vi "generateTimeStamp.vi"(8 "error in (no error)":errorcluster, 11 "FileNeologist in":refnum<class "FileNeologist.lvclass">) -> (0 "error out":errorcluster, 3 "FileNeologist out":refnum<class "FileNeologist.lvclass">)   [LabVIEW 2009, in "Tools.lvlib" / "Filing.lvlib" / "FileNeologist.lvclass"]
uses:
  FileNeologist.lvclass
  FileNeologist.lvclass/FileNeologist.ctl
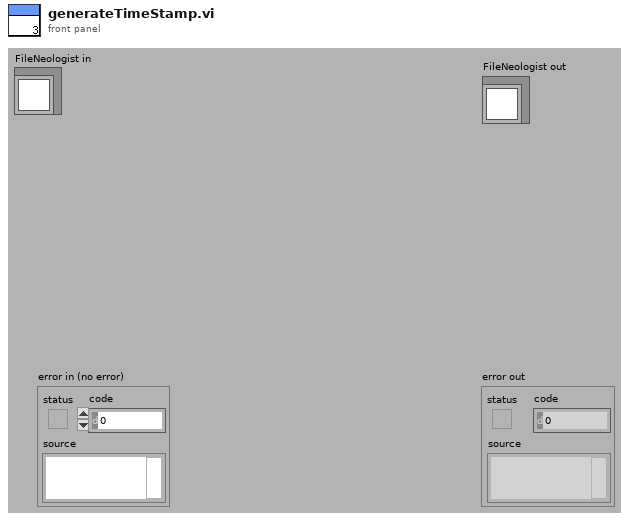
[diagram p1: front panel]
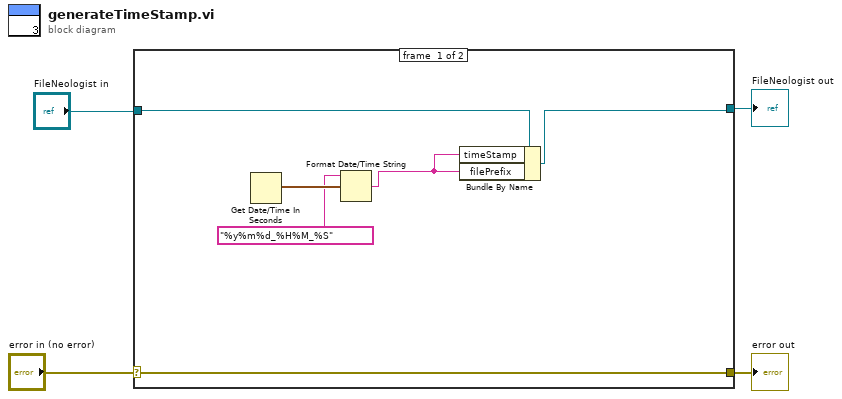
[diagram p0: block diagram]
diagram:
  n1 = case shown="No Error" "error in (no error)" {
    selector: "error in (no error)" -> [w10 w12]
    tunnel: [w10 w12] -> w3
    tunnel: [w6 w11] -> w2
    tunnel: "FileNeologist in" -> [w7 w11]
    frame #0 {
      n2 = Get Date/Time In Seconds() -> (seconds since 1Jan1904=w9:timestamp)
      n3 = Format Date/Time String(time format string (%c)="%y%m%d_%H%M_%S", seconds (now)=w9) -> (date/time string=w5:string)  [unwired: 1 in]
      n4 = Bundle By Name(cluster=w7, "timeStamp"=w5, "filePrefix"=w5) -> (w6:refnum<class "FileNeologist.lvclass">)
    }
    frame #1 {
    }
  }
  "error out" <- w3
  "FileNeologist out" <- w2
